vi "Find path stem for EP.vi"(0 "Node of path stem.":string) -> (1 "Path stem.":path, 2 "PASS/FAIL":bool)   [LabVIEW 2010]
panel:
  # "Inputs:"
  # "Outputs:"
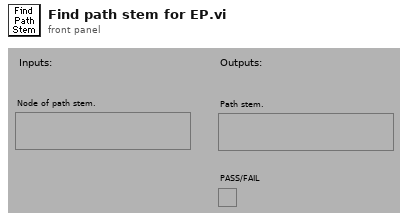
[diagram p1: front panel]
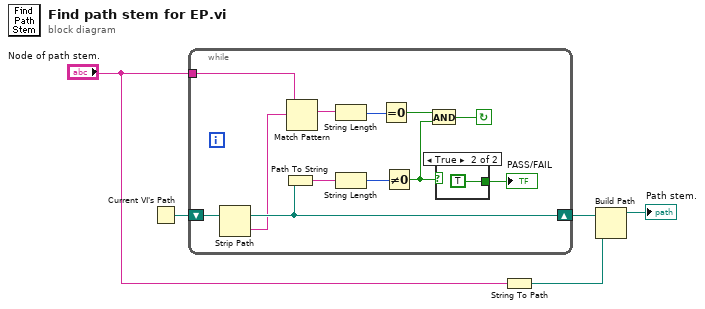
[diagram p0: block diagram]
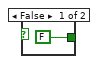
[diagram p2: hidden frame]
diagram:
  n1 = Current VI's Path() -> (path=w2:path)
  n2 = while {
    tunnel: "Node of path stem." -> [w9]
    shift-left: w2 -> [w17]
    shift-right: [w14] -> w5
    stop <- w10 continue-if-true
    n3 = Strip Path(path=w17) -> (stripped path=w14:path, name=w7:string)
    n4 = Path To String(path=w14) -> (string=w16:string)
    n5 = Match Pattern(string=w7, regular expression=w9) -> (match substring=w8:string)  [unwired: 4 out]
    n6 = String Length(string=w8) -> (length=w12:i32)
    n7 = String Length(string=w16) -> (length=w15:i32)
    n8 = Equal To 0?(x=w12) -> (x = 0?=w6:bool)
    n9 = Not Equal To 0?(x=w15) -> (x != 0?=w11:bool)
    n10 = And(x=w6, y=w11) -> (x .and. y?=w10:bool)
    n11 = case shown="True" w11 {
      tunnel: [FALSE TRUE] -> w13
      frame False {
      }
      frame True {
      }
    }
    "PASS/FAIL" <- w13
  }
  n12 = String To Path(string="Node of path stem.") -> (path=w3:path)
  n13 = Build Path(base path=w5, name or relative path=w3) -> (appended path=→"Path stem.":path)
